vi "Yscaling_FBL.vi"(8 "Nano Z Read":dbl, 9 "Current Maxed?":bool, 10 "Y":dbl, 11 "Plane Height":dbl) -> (3 "y scaled (m)":dbl, 4 "Zpos Graph (nm)":cluster{dbl, "function return":dbl})   [LabVIEW 2019]
uses:
  GlobalClicksHeight_FBL.vi
  <userlib>/HapticSTM/HapticSTM.lvlib
panel:
  out "Testoutput":dbl
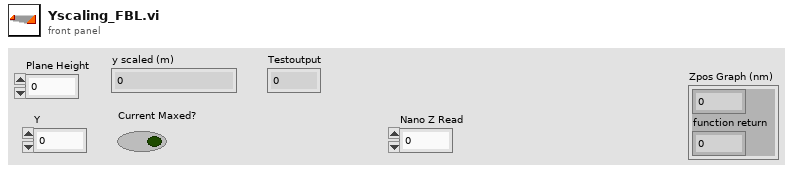
[diagram p1: front panel]
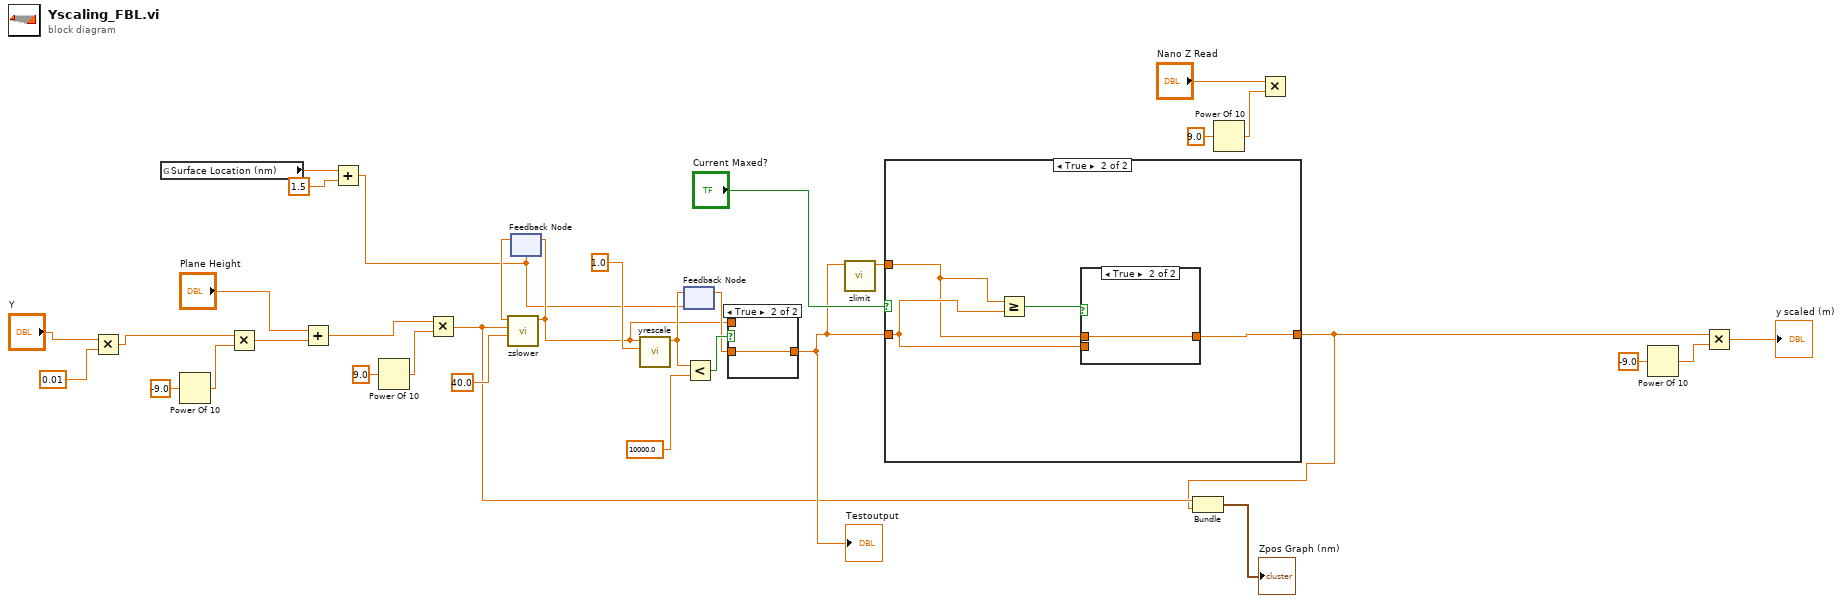
[diagram p0: block diagram]
diagram:
  n1 = Multiply(x="Y", y=0.01) -> (x*y=w29:dbl)
  n2 = global read "GlobalClicksHeight_FBL.vi" "Surface Location (nm)"() -> (w2:dbl)
  n3 = Power Of 10(x=-9.0) -> (10^x=w28:dbl)
  n4 = Multiply(x=w29, y=w28) -> (x*y=w30:dbl)
  n5 = Add(x="Plane Height", y=w30) -> (x+y=w33:dbl)
  n6 = Add(x=w2, y=1.5) -> (x+y=w1:dbl)
  n7 = Power Of 10(x=9.0) -> (10^x=w32:dbl)
  n8 = Multiply(x=w33, y=w32) -> (x*y=w7:dbl)
  n9 = feedback #1(w1) -> (w9:dbl)
  n10 = call <userlib>:"zslower.vi"("maxvel"=40.0, "labview_zpos_write"=w7, "nanonis_zpos_read"=w9) -> ("function return"=w4:dbl)  [unwired: 8 in]
  n11 = feedback-in #1(w4) -> ()
  n12 = call <userlib>:"yrescale.vi"("scalingfactor"=1.0, "ylabview"=w4) -> ("function return"=w5:dbl)  [unwired: 9 in]
  n13 = feedback-in #2(w5) -> ()
  n14 = feedback #2(w1) -> (w14:dbl)
  n15 = Less?(x=w5, y=10000.0) -> (x < y?=w15:bool)
  n16 = case shown="True" w15 {
    tunnel: [w34 w35] -> w17
    tunnel: w14 -> [_ w35]
    tunnel: w4 -> [w34 _]
    frame False {
    }
    frame True {
    }
  }
  "Testoutput" <- w17
  n17 = call <userlib>:"zlimit.vi"("yscaledinput"=w17) -> ("function return"=w18:dbl)  [unwired: 10 in]
  n18 = case shown="True" "Current Maxed?" {
    tunnel: [w36 w40] -> w6
    tunnel: w17 -> [w36 w38]
    tunnel: w18 -> [_ w37]
    frame False {
    }
    frame True {
      n19 = Greater Or Equal?(x=w37, y=w38) -> (x >= y?=w39:bool)
      n20 = case shown="True" w39 {
        tunnel: w37 -> [_ w42]
        tunnel: [w41 w42] -> w40
        tunnel: w38 -> [w41 _]
        frame False {
        }
        frame True {
        }
      }
    }
  }
  n21 = Bundle(w7, "function return"=w6) -> (→"Zpos Graph (nm)":cluster{dbl, "function return":dbl})  [unwired: 1 in]
  n22 = Power Of 10(x=9.0) -> (10^x=w13:dbl)
  n23 = Multiply(x="Nano Z Read", y=w13) -> ()  [unwired: 1 out]
  n24 = Power Of 10(x=-9.0) -> (10^x=w21:dbl)
  n25 = Multiply(x=w6, y=w21) -> (x*y=→"y scaled (m)":dbl)
